vi "ConvertHexStringtoNormal.vi"(1 "Hex String":string="Hello World!") -> (0 "Normal String":string)   [LabVIEW 2012, in "NFC Driver.lvlib"]
doc: "This VI converts a raw HEX string into it's ASCII representation"
uses:
  NFC Driver.lvlib
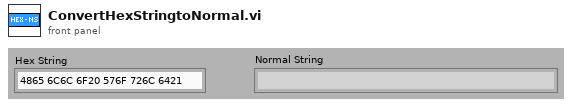
[diagram p1: front panel]
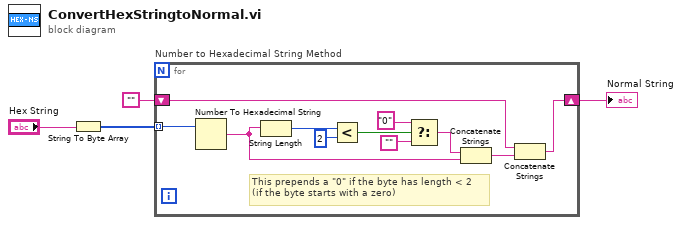
[diagram p0: block diagram]
diagram:
  n1 = String To Byte Array(string="Hex String") -> (unsigned byte array=w1:u8[])
  n2 = for "Number to Hexadecimal String Method" {
    shift-right: [w15] -> w3
    shift-left: "" -> [w5]
    tunnel: w1 -> [w6] mode=indexing
    # "This prepends a \"0\" if the byte has length < 2\n(if the byte starts with a zero)"
    n3 = Number To Hexadecimal String(2:w6) -> (0:w8:string)  [unwired: 1 in]
    n4 = String Length(string=w8) -> (length=w14:i32)
    n5 = Less?(x=w14, y=2) -> (x < y?=w12:bool)
    n6 = Select(t="0", s=w12, f="") -> (s? t:f=w9:string)
    n7 = Concatenate Strings(w9, w8) -> (w7:string)
    n8 = Concatenate Strings(w5, w7) -> (w15:string)
  }
  "Normal String" <- w3
